vi "display module.vi"(7 "Action":enum16{"Init", "display", "Uninit"}(ring)=enum."Uninit", 8 "error in":errorcluster, 11 "data in":sgl[][](array[numeric])) -> (0 "error out":errorcluster, 2 "Image":T1(plugin-control), 3 "display successful?":bool)   [LabVIEW 2018]
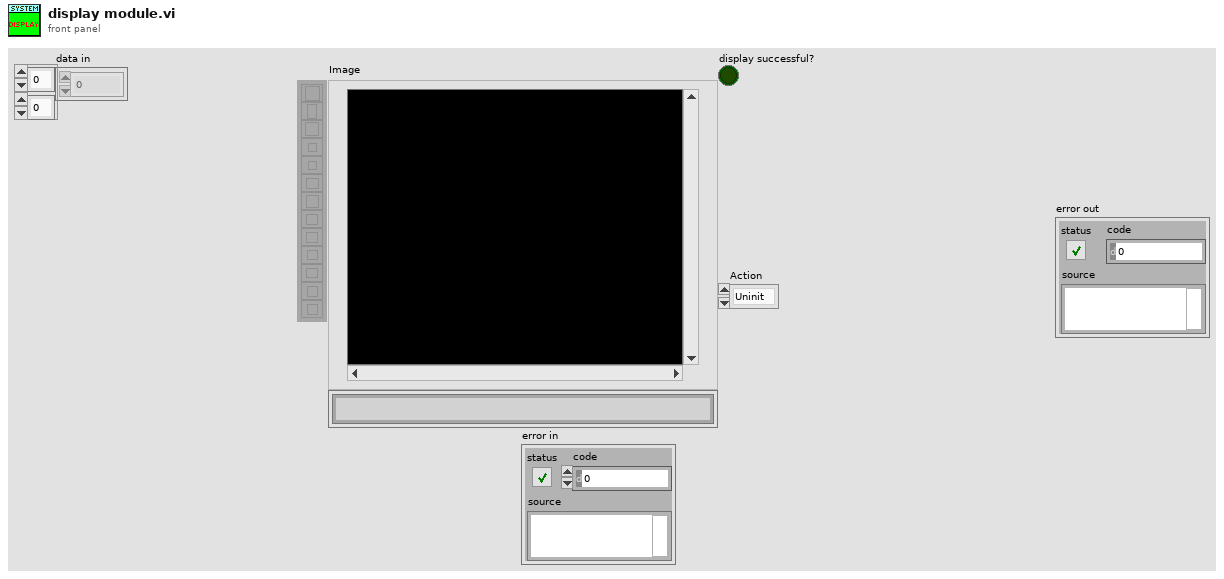
[diagram p1: front panel]
types:
  T1 = typedef "IMAQ Image.ctl" = refnum<image>
  T2 = typedef "Image Type" = u32
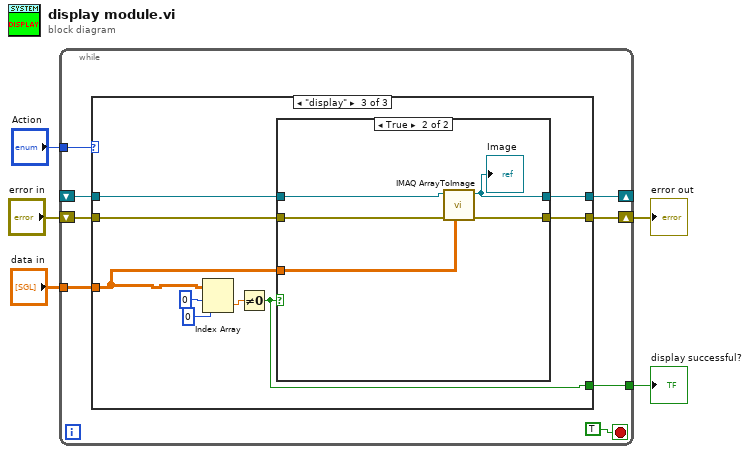
[diagram p0: block diagram]
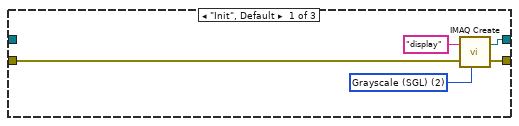
[diagram p2: hidden frame]
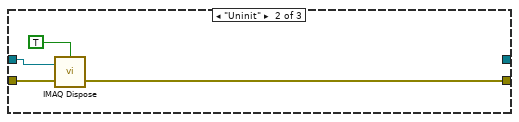
[diagram p3: hidden frame]
diagram:
  n1 = while {
    tunnel: "Action" -> [w13]
    shift-right: [w12] -> _
    shift-left: _ -> [w11]
    shift-right: [w9] -> w3
    shift-left: "error in" -> [w10]
    tunnel: [w7] -> w2
    tunnel: "data in" -> [w6]
    stop <- TRUE stop-if-true
    n2 = case shown="\"display\"" w13 {
      tunnel: [w18 _ w31] -> w12
      tunnel: w11 -> [_ w22 w30]
      tunnel: w10 -> [w17 w21 w29]
      tunnel: [w16 w20 w28] -> w9
      tunnel: [_ _ w25] -> w7
      tunnel: w6 -> [_ _ w24]
      frame "Init", Default {
        w14 = T2 2 items=["Grayscale (U8)", "Grayscale (I16)", "Grayscale (SGL)", "Complex (CSG)", "RGB (U32)", "HSL (U32)", "RGB (U64)", "Grayscale (U16)"] ("Image Type")
        n3 = call "IMAQ Create"("Image Name"="display", "Image Type"=w14, "error in (no error)"=w17) -> ("New Image"=w18:T1, "error out"=w16:errorcluster)  [unwired: 2 in]
      }
      frame "Uninit" {
        n4 = call "IMAQ Dispose"("All Images? (No)"=TRUE, "Image"=w22, "error in (no error)"=w21) -> ("error out"=w20:errorcluster)  [unwired: 3 in]
      }
      frame "display" {
        n5 = Index Array(array=w24, index (row)=0 ("index"), index (col)=0 ("disabled index (col)")) -> (element=w26:sgl)
        n6 = Not Equal To 0?(x=w26) -> (x != 0?=w25:bool)
        n7 = case shown="True" w25 {
          tunnel: [w33 w38] -> w31
          tunnel: [w32 w37] -> w28
          tunnel: w30 -> [w33 w35]
          tunnel: w29 -> [w32 w36]
          tunnel: w24 -> [_ w34]
          frame False {
          }
          frame True {
            n8 = call "IMAQ ArrayToImage"("Image Pixels (Float)"=w34, "error in (no error)"=w36, "Image"=w35) -> ("error out"=w37:errorcluster, "Image Out"=w38:T1)  [unwired: 7 in]
            "Image" <- w38
          }
        }
      }
    }
  }
  "error out" <- w3
  "display successful?" <- w2
